vi "TSM Relays to Relay Configuration.vi"(0 "TSM Context":T4, 5 "Relay/Action Connections":T1[](array[typedef]) {"Relay Action" items=["Open Relay"=20, "Close Relay"=21]}, 11 "error in":errorcluster) -> (4 "Relay Configuration Out":T3 {"Relay Action Configuration"."Relay Action" items=["Open Relay"=20, "Close Relay"=21]}, 15 "error out":errorcluster)   [LabVIEW 2019]
doc: "Populates the Relay Configuration cluster for the selected relay/action connections. This VI can be used to implement a relay configuration (set of mappings between relay(s) and positions) within a test code module."
uses:
  <vilib>/NI_TestStand_SemiconductorModule/NI_TestStand_Semiconductor_Module.lvlibp/PinMap/General/SemiconductorModuleContext.ctl
  TSM Relay Configuration.ctl
  TSM Relay to Action Map.ctl
  <vilib>/NI_TestStand_SemiconductorModule/NI_TestStand_Semiconductor_Module.lvlibp/1abvi3w/instr.lib/niSwitch/niswitch.llb/niSwitch Relay Action.ctl
  <vilib>/NI_TestStand_SemiconductorModule/NI_TestStand_Semiconductor_Module.lvlibp
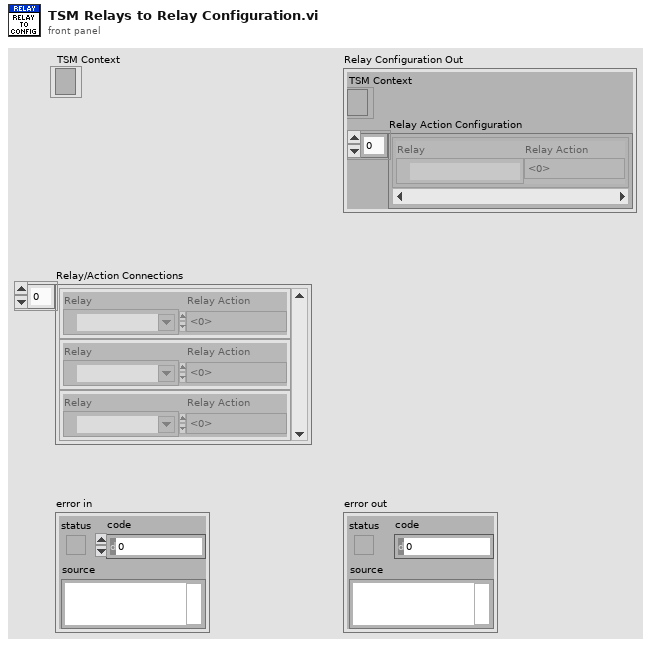
[diagram p1: front panel]
types:
  T1 = typedef "TSM Relay to Action Map.ctl" = cluster{"Relay":tag, "Relay Action":T2}
  T2 = typedef "NI_TestStand_Semiconductor_Module.lvlibp/niSwitch Relay Action.ctl" = i32
  T3 = typedef "TSM Relay Configuration.ctl" = cluster{"TSM Context":T4, "Relay Action Configuration":T1[]}
  T4 = typedef "NI_TestStand_Semiconductor_Module.lvlibp/SemiconductorModuleContext.ctl" = refnum<k7>
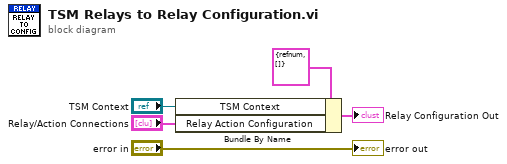
[diagram p0: block diagram]
diagram:
  n1 = Bundle By Name(cluster=T3 {"TSM Context"=refnum, "Relay Action Configuration"=[]} ("TSM SSC Relay Configuration Out 2"), "TSM Context"="TSM Context", "Relay Action Configuration"="Relay/Action Connections") -> (→"Relay Configuration Out":T3)
  "error out" <- "error in"
